vi "NtfyLvFpga_SUB_InTimeRange_ProhibitTimeHour.vi"(9 "Time Range":T1={"chk enable"=TRUE, "start hour"=23, "end hour"=6}, 11 "timestamp":timestamp format="%<%H:%M:%S>T") -> (2 "InRange":bool)   [LabVIEW 2013]
panel:
  # "timestamp が指定時間帯(Time Range)かどうか?"
  # "timestamp 未配線の場合は、現在時間で判定します。"
  # "6:00 to 9:00 の場合は、6:00から9:00までが範囲内。\n23:00 to 6:00 の場合は、23:00から次の日の6:00までが範囲内。\nstart hour と end hour が同じ場合は無効、常に範囲外と判断される。"
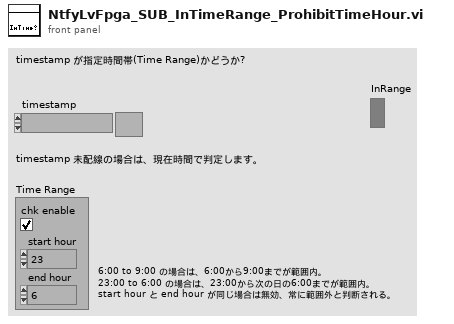
[diagram p1: front panel]
types:
  T1 = cluster{"chk enable":bool, "start hour":u8, "end hour":u8}
  T2 = typedef "LVDateTimeRec.ctl" = cluster{"小数秒":dbl, "秒":i32, "分":i32, "時間":i32, "日":i32, "月":i32, "年":i32, "曜日":i32, "年間通算日":i32, "DST":i32}
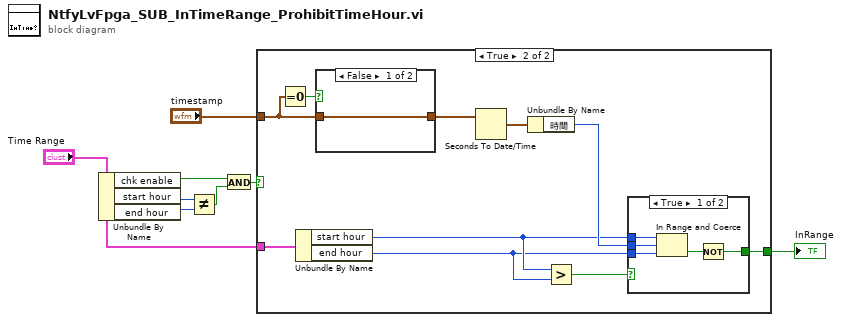
[diagram p0: block diagram]
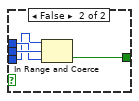
[diagram p3: hidden frame]
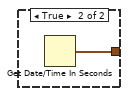
[diagram p4: hidden frame]
diagram:
  n1 = Unbundle By Name("Time Range") -> ("chk enable"=w5:bool, "start hour"=w7:u8, "end hour"=w6:u8)
  n2 = Not Equal?(x=w7, y=w6) -> (x != y?=w1:bool)
  n3 = And(x=w5, y=w1) -> (x .and. y?=w4:bool)
  n4 = case shown="TRUE" w4 {
    tunnel: "timestamp" -> [_ w17]
    tunnel: "Time Range" -> [_ w14]
    tunnel: [_ w9] -> w2
    frame False {
    }
    frame True {
      n5 = Equal To 0?(x=w17) -> (x = 0?=w18:bool)
      n6 = Unbundle By Name(w14) -> ("start hour"=w11:u8, "end hour"=w10:u8)
      n7 = case shown="FALSE" w18 {
        tunnel: w17 -> [w28 _]
        tunnel: [w28 w29] -> w16
        frame False {
        }
        frame True {
          n8 = Get Date/Time In Seconds() -> (seconds since 1Jan1904=w29:timestamp)
        }
      }
      n9 = Seconds To Date/Time(time stamp (now)=w16) -> (date time rec=w15:T2)  [unwired: 1 in]
      n10 = Unbundle By Name(w15) -> ("時間"=w12:i32)
      n11 = Greater?(x=w11, y=w10) -> (0:w13:bool)
      n12 = case shown="TRUE" w13 {
        tunnel: w12 -> [w23 w27]
        tunnel: w11 -> [w22 w26]
        tunnel: w10 -> [w21 w25]
        tunnel: [w19 w24] -> w9
        frame True {
          n13 = In Range and Coerce(upper limit=w22, x=w23, lower limit=w21) -> (In Range?=w20:bool)  [unwired: 1 out]
          n14 = Not(x=w20) -> (.not. x?=w19:bool)
        }
        frame False {
          n15 = In Range and Coerce(upper limit=w25, x=w27, lower limit=w26) -> (In Range?=w24:bool)  [unwired: 1 out]
        }
      }
    }
  }
  "InRange" <- w2
